vi "Pos.vi"(3 "error in":errorcluster, 5 "name or relative path":path) -> (0 "error out":errorcluster, 2 "output cluster":T1)   [LabVIEW 2025]
panel:
  out "Sw":i32
  out "Yw":i32
  out "Xw":i32
  out "Sy":i32
  out "Yy":i32
  out "Xy":i32
  out "Sr":i32
  out "Yr":i32
  out "Xr":i32
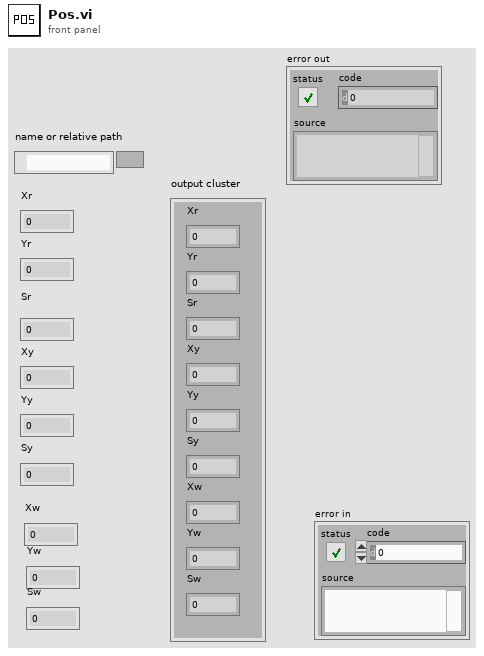
[diagram p1: front panel]
types:
  T1 = cluster{"Xr":i32, "Yr":i32, "Sr":i32, "Xy":i32, "Yy":i32, "Sy":i32, "Xw":i32, "Yw":i32, "Sw":i32}
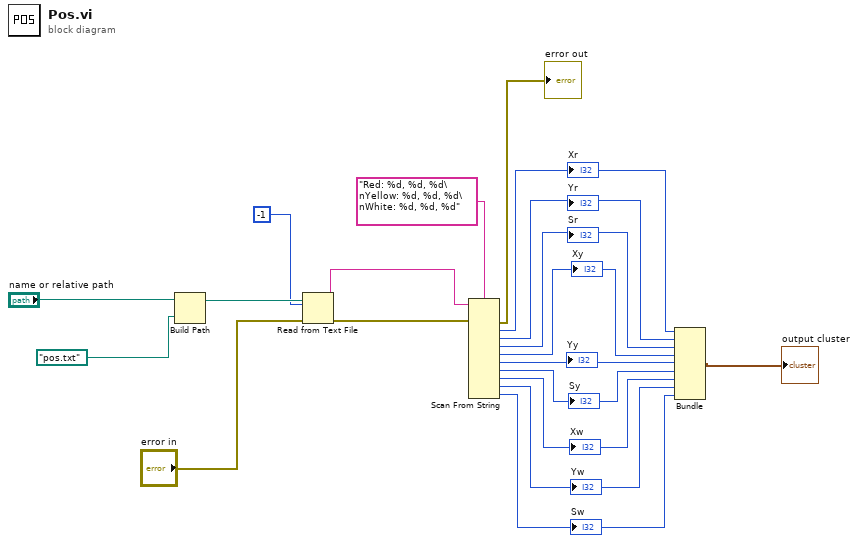
[diagram p0: block diagram]
diagram:
  n1 = Build Path(base path="name or relative path", name or relative path=path "pos.txt") -> (appended path=w18:path)
  n2 = Read from Text File(file (use dialog)=w18, count=-1, error in="error in") -> (text=w6:string, error out=w4:errorcluster)  [unwired: 1 in, 2 out]
  n3 = Scan From String(format string="Red: %d, %d, %d\nYellow: %d, %d, %d\nWhite: %d, %d, %d", input string=w6, error in=w4) -> (error out=→"error out":errorcluster, output 1=w17:i32, output 2=w16:i32, output 3=w15:i32, output 4=w14:i32, output 5=w13:i32, output 6=w12:i32, output 7=w10:i32, output 8=w9:i32, output 9=w8:i32)  [unwired: 10 in, 2 out]
  "Xr" <- w17
  "Yr" <- w16
  "Sr" <- w15
  "Xy" <- w14
  "Yy" <- w13
  "Sy" <- w12
  "Xw" <- w10
  "Yw" <- w9
  "Sw" <- w8
  n4 = Bundle("Xr"=w17, "Yr"=w16, "Sr"=w15, "Xy"=w14, "Yy"=w13, "Sy"=w12, "Xw"=w10, "Yw"=w9, "Sw"=w8) -> (→"output cluster":T1)  [unwired: 1 in]
